vi "set_frequency.vi"(8 "error in":errorcluster, 9 "Variable Names":string[](array[string]), 10 "Variable Values":dbl[](array[numeric]) format="%.2f", 11 "RF Generator settings":T1) -> (0 "error out":errorcluster)   [LabVIEW 2012, in "HP8662A_RF_Generator.lvclass"]
uses:
  HP8662A_RF_Generator.lvclass
  <vilib>/Instr/_visa.llb/GPIB Status Boolean Array.ctl
  RF_Generator_settings.ctl
  <vilib>/gmath/NI_Gmath.lvlib
  GPIB.lvclass
panel:
  out "status":T2
  out "GPIB channel #":string
  out "resulting string":string
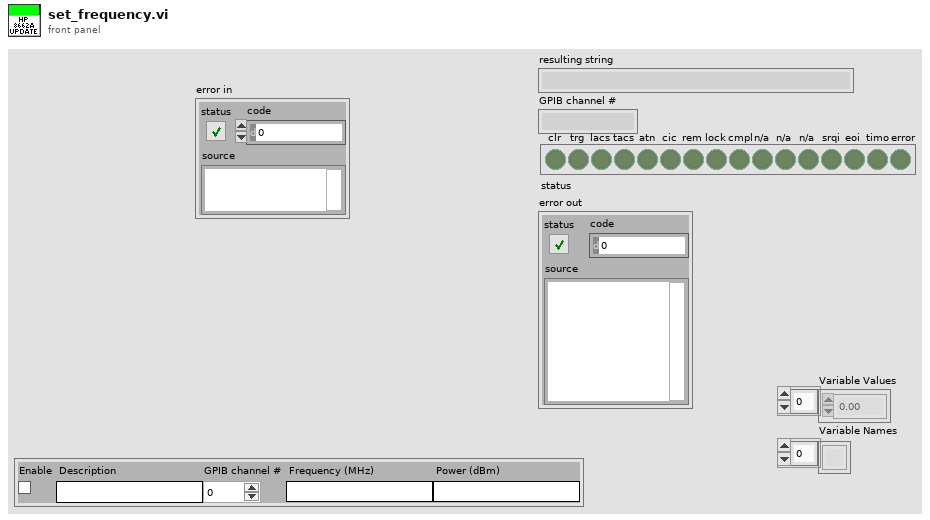
[diagram p1: front panel]
types:
  T1 = typedef "GPIB.lvclass/RF_Generator_settings.ctl" = cluster{"Enable":bool, "Description":string, "GPIB channel #":u8, "Frequency (MHz)":string, "Power (dBm)":string}
  T2 = typedef "GPIB Status Boolean Array.ctl" = bool[]
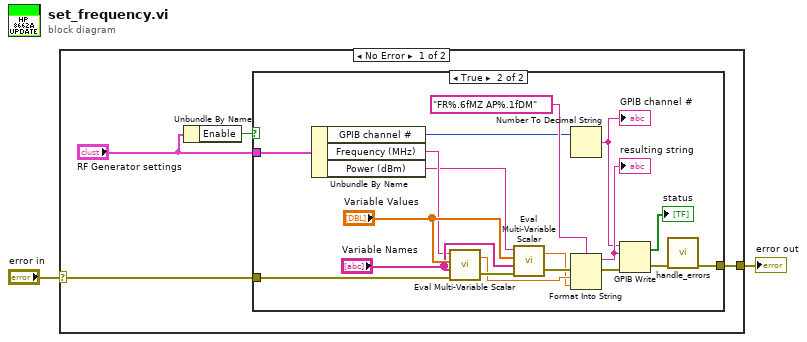
[diagram p0: block diagram]
diagram:
  n1 = case shown="No Error" "error in" {
    selector: "error in" -> [w4 w26]
    tunnel: [w3 w26] -> w1
    frame No Error {
      n2 = Unbundle By Name("RF Generator settings") -> ("Enable"=w5:bool)
      n3 = case shown="True" w5 {
        tunnel: "RF Generator settings" -> [_ w14]
        tunnel: w4 -> [w7 w12]
        tunnel: [w7 w13] -> w3
        frame False {
        }
        frame True {
          n4 = Unbundle By Name(w14) -> ("GPIB channel #"=w15:u8, "Frequency (MHz)"=w17:string, "Power (dBm)"=w16:string)
          n5 = call <vilib>:"Eval Multi-Variable Scalar.vi"("error in (no error)"=w12, "Variables"="Variable Names", "X Values"="Variable Values", "formula"=w17) -> ("error out"=w11:errorcluster, "y value"=w9:dbl)
          n6 = call <vilib>:"Eval Multi-Variable Scalar.vi"("error in (no error)"=w11, "Variables"="Variable Names", "X Values"="Variable Values", "formula"=w16) -> ("error out"=w10:errorcluster, "y value"=w8:dbl)
          n7 = Number To Decimal String(number=w15) -> (decimal integer string=w23:string)  [unwired: 1 in]
          "GPIB channel #" <- w23
          n8 = Format Into String(format string="FR%.6fMZ AP%.1fDM", error in=w10, w9, w8) -> (resulting string=w24:string, error out=w21:errorcluster)  [unwired: 1 in]
          "resulting string" <- w24
          n9 = GPIB Write(0:w23, 1:w24, 3:w21) -> (5:→"status":bool[], 6:w20:errorcluster)  [unwired: 2 in]
          n10 = call "handle_errors.vi"("error in (no error)"=w20) -> ("error out"=w13:errorcluster)  [unwired: 10 in]
        }
      }
    }
    frame Error {
    }
  }
  "error out" <- w1
